vi "Open Hardware.vi"(8 "error in (no error)":errorcluster, 11 "Instrument in":refnum<class "Instrument.lvclass">) -> (0 "error out":errorcluster, 3 "Instrument out":refnum<class "Instrument.lvclass">)   [LabVIEW 2019, in "Instrument.lvclass"]
doc: "Override to <b>open</b> a connection to your instrument."
uses:
  Instrument.lvclass
  Instrument.lvclass/Instrument.ctl
  subsystems/HAL/HAL.lvclass
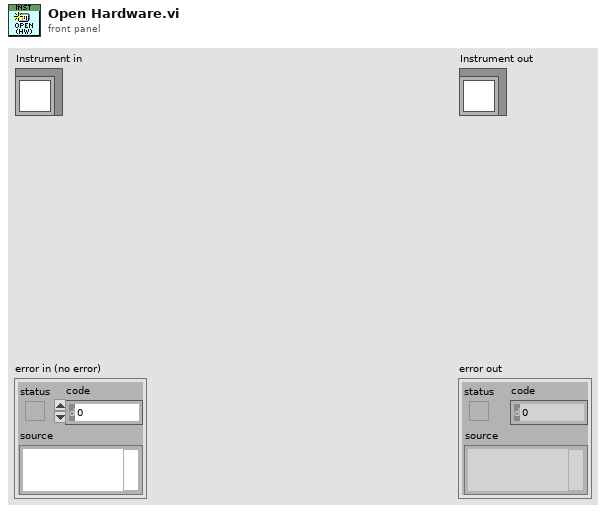
[diagram p1: front panel]
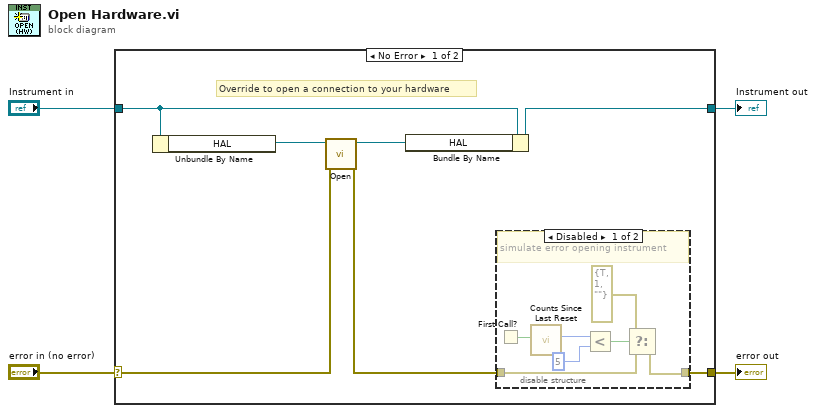
[diagram p0: block diagram]
diagram:
  n1 = case shown="No Error" "error in (no error)" {
    selector: "error in (no error)" -> [w9 w21]
    tunnel: [w11 w21] -> w3
    tunnel: [w7 w20] -> w1
    tunnel: "Instrument in" -> [w6 w20]
    frame No Error {
      # "Override to open a connection to your hardware"
      n2 = Unbundle By Name(w6) -> ("HAL"=w10:refnum<class "HAL.lvclass">)
      n3 = call-dynamic "Open.vi"("error in (no error)"=w9, "HAL in"=w10) -> ("error out"=w8:errorcluster, "HAL out"=w5:refnum<class "HAL.lvclass">)  [unwired: 8 in]
      n4 = Bundle By Name(cluster=w6, "HAL"=w5) -> (w7:refnum<class "Instrument.lvclass">)
      n5 = disable-structure shown="Disabled" {
        disable-tunnel: w8 -> [w17 w19]
        disable-tunnel: [w16 w19] -> w11
        frame Disabled {
          # "simulate error opening instrument"
          n6 = First Call?() -> (First Call?: T/F=w13:bool)
          n7 = call "Counts Since Last Reset.vi"("Reset (F)"=w13) -> ("counter"=w12:u32)  [unwired: 5 in, 1 out]
          n8 = Less?(x=w12, y=u32 5 ("x")) -> (x < y?=w18:bool)
          n9 = Select(t=errorcluster {"status"=TRUE, "code"=1, "source"=""}, s=w18, f=w17) -> (s? t:f=w16:errorcluster)
        }
        frame Enabled {
        }
      }
    }
    frame Error {
    }
  }
  "error out" <- w3
  "Instrument out" <- w1
